vi "PointRotation.vi"(2 "Rotation (deg)":dbl, 3 "Y Points":dbl[](array[numeric]), 4 "X Points":dbl[](array[numeric])) -> (0 "Y' Points":dbl[](array[numeric]), 1 "X' Points":dbl[](array[numeric]))   [LabVIEW 2016]
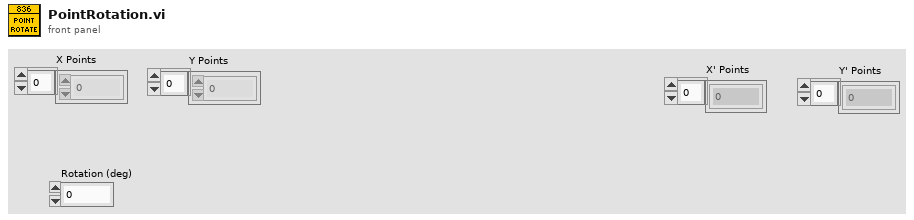
[diagram p1: front panel]
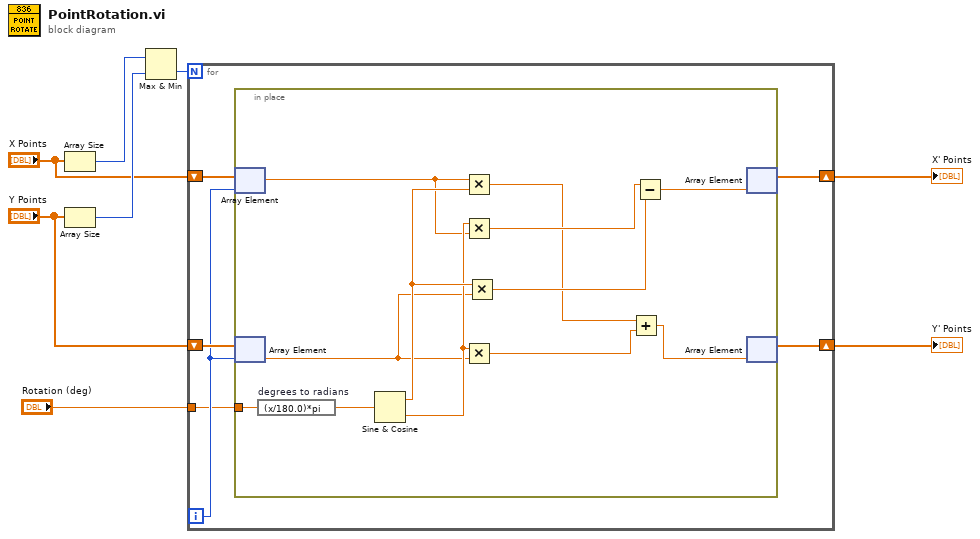
[diagram p0: block diagram]
diagram:
  n1 = Array Size(array="X Points") -> (size(s)=w8:i32)
  n2 = Array Size(array="Y Points") -> (size(s)=w7:i32)
  n3 = Max & Min(x=w8, y=w7) -> (min(x,y)=w6:i32)  [unwired: 1 out]
  n4 = for {
    N: w6 -> [_]
    tunnel: "Rotation (deg)" -> [w11]
    shift-right: [w10] -> w2
    shift-left: "X Points" -> [w14]
    shift-right: [w9] -> w1
    shift-left: "Y Points" -> [w13]
    i -> [w12]
    n5 = in-place {
      in-place-border: w11 -> [w16]
      n6 = in-place-array #1(w14, w12) -> (w24:dbl)
      n7 = in-place-array #2(w13, w12) -> (w23:dbl)
      n8 = expression code="(x/180.0)*pi" "degrees to radians"(w16) -> (w15:dbl)
      n9 = Sine & Cosine(0:w15) -> (1:w26:dbl, 2:w25:dbl)
      n10 = Multiply(x=w24, y=w26) -> (x*y=w20:dbl)
      n11 = Multiply(x=w25, y=w24) -> (x*y=w22:dbl)
      n12 = Multiply(x=w25, y=w23) -> (x*y=w19:dbl)
      n13 = Multiply(x=w26, y=w23) -> (x*y=w21:dbl)
      n14 = Add(x=w20, y=w19) -> (x+y=w18:dbl)
      n15 = Subtract(x=w22, y=w21) -> (x-y=w17:dbl)
      n16 = in-place-array #1(w17) -> (w10:dbl[])  [unwired: 1 out]
      n17 = in-place-array #2(w18) -> (w9:dbl[])  [unwired: 1 out]
    }
  }
  "X' Points" <- w2
  "Y' Points" <- w1
